vi "Msg.vi"(7 "Actor in":refnum<class "Actor.lvclass">, 11 "Stop Msg in":refnum<class "Destroy Msg.lvclass">) -> (0 "error out":errorcluster, 2 "Destroy Self?":bool, 5 "Actor out":refnum<class "Actor.lvclass">)   [LabVIEW 2021, in "Destroy.lvlib" / "Destroy Msg.lvclass"]
uses:
  Destroy Msg.lvclass
  AAM/Actor/Actor.lvclass
  Destroy/Destroy.lvclass
  Destroy Msg.lvclass/Destroy Msg.ctl
  4f9a6ab2-8004-4bc5-8151-3b11a1296234.vi
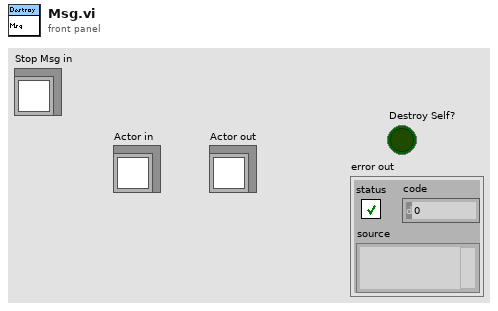
[diagram p1: front panel]
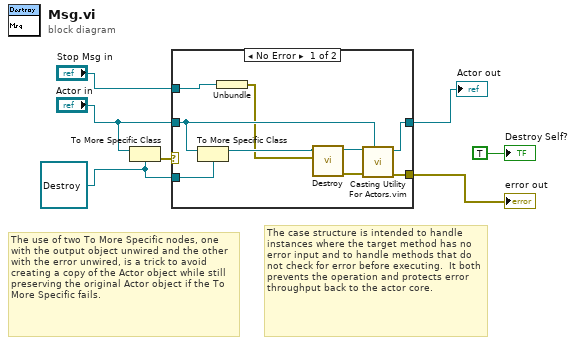
[diagram p0: block diagram]
diagram:
  w2 = refnum<class "Destroy.lvclass"> refnum ("Destroy.lvlib:Destroy.lvclass")
  # "The use of two To More Specific nodes, one with the output object unwired and the other with the error unwired, is a trick to avoid creating a copy of the Actor object while still preserving the original Actor object if the To More Specific fails."
  # "The case structure is intended to handle instances where the target method has no error input and to handle methods that do not check for error before executing.  It both prevents the operation and protects error throughput back to the actor core."
  n1 = To More Specific Class(target class=w2, reference="Actor in") -> (error out=w7:errorcluster)  [unwired: 1 in, 1 out]
  n2 = case shown="No Error" w7 {
    selector: w7 -> [_ w18]
    tunnel: [w13 w18] -> w6
    tunnel: [w14 w17] -> w3
    tunnel: "Actor in" -> [w15 w17]
    tunnel: w2 -> [w16 _]
    tunnel: "Stop Msg in" -> [w9 _]
    frame No Error {
      n3 = To More Specific Class(target class=w16, reference=w15) -> (specific class reference=w10:refnum<class "Destroy.lvclass">)  [unwired: 1 in, 1 out]
      n4 = Unbundle(w9) -> (w8:errorcluster)
      n5 = call-dynamic "Destroy.vi"("Error"=w8, "Destroy in"=w10) -> ("error out"=w11:errorcluster, "Destroy out"=w12:refnum<class "Destroy.lvclass">)  [unwired: 8 in]
      n6 = call "Casting Utility For Actors.vim"("type"=w15, "error in (no error)"=w11, "Actor in"=w12) -> ("error out"=w13:errorcluster, "Actor out"=w14:refnum<class "Actor.lvclass">)  [unwired: 7 in]
    }
    frame Error {
      # "If type check fails, pass the original object out again."
    }
  }
  "error out" <- w6
  "Actor out" <- w3
  "Destroy Self?" <- TRUE ("Destroy Self")
